vi "MainBootstrap.vi"() -> ()   [LabVIEW 2017]
uses:
  <vilib>/NI/Software Watchdog/Pound/Pound.lvclass
  <vilib>/addons/BlinkProcess/controls/mode.ctl
  <vilib>/addons/InsightCM/Devices/Shared/Common/Controller/controls/operations.ctl
  <vilib>/addons/TraceLogger/TraceLogger.lvlib
  <vilib>/addons/Qbus/Qbus.lvclass
  <vilib>/addons/InsightCM/Devices/Shared/Common/ServerComm/ServerComm.lvlib
  <vilib>/addons/TimerProcess/TimerProcess.lvlib
  <vilib>/addons/BlinkProcess/BlinkProcess.lvlib
  <vilib>/addons/InsightCM/Devices/Shared/Common/TracePointDisplay/TracePointDisplay.lvlib
  <vilib>/addons/InsightCM/Devices/Shared/Common/Controller/Controller.lvlib
  <vilib>/addons/InsightCM/Utilities/GlobalConfiguration/GlobalConfiguration.lvlib
panel:
  out "Log":string
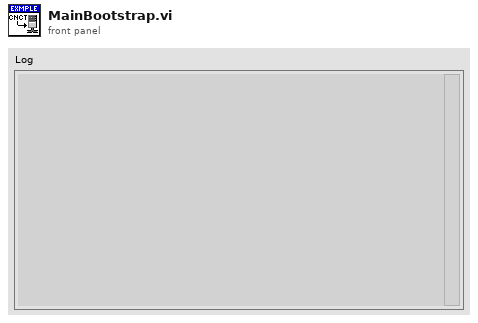
[diagram p1: front panel]
types:
  T1 = typedef "BlinkProcess.lvlib/mode.ctl" = enum16{"Normal", "Error", "On", "Off", "Custom"}
  T2 = typedef "Controller.lvlib/operations.ctl" = enum16{"Unknown", "Startup", "Expected Shutdown"}
  T3 = typedef "ServerComm.lvlib/ConnectionStatus.ctl" = enum16{"Offline", "NotAuthorized", "Online"}
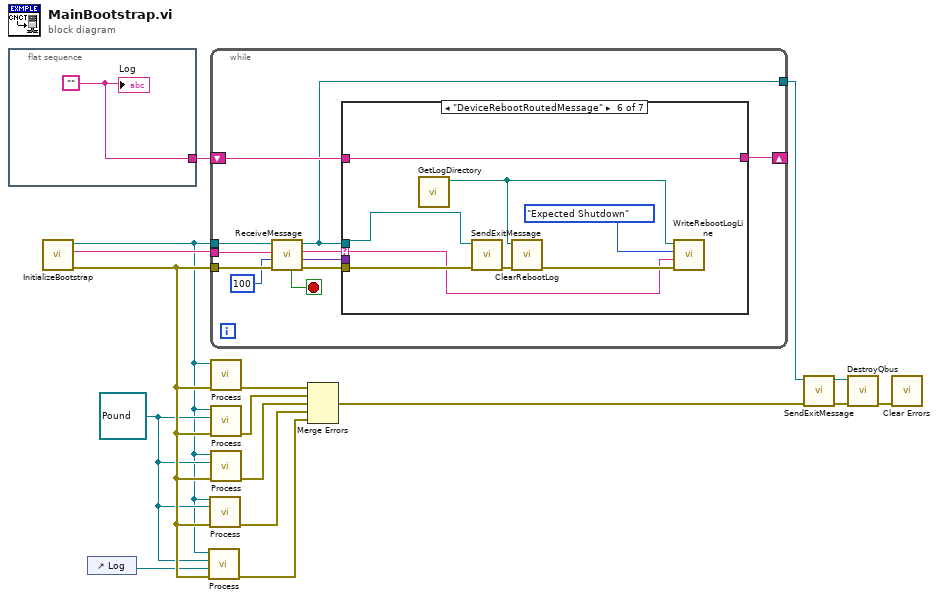
[diagram p0: block diagram]
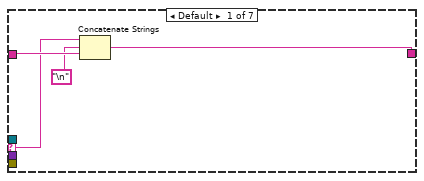
[diagram p2: hidden frame]
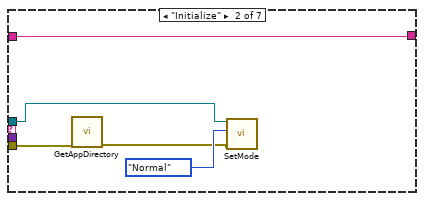
[diagram p3: hidden frame]
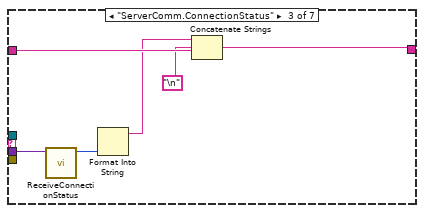
[diagram p4: hidden frame]
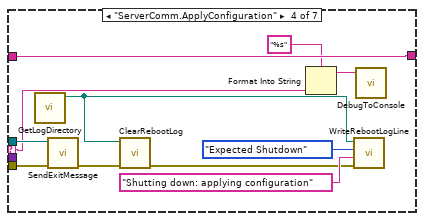
[diagram p5: hidden frame]
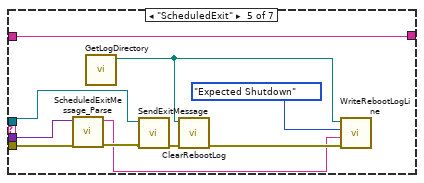
[diagram p6: hidden frame]
diagram:
  w4 = refnum<class "Pound.lvclass"> refnum ("Pound in")
  n1 = flat-sequence {
    tunnel: [w16] -> w13
    frame #0 {
      w16 = ""
      "Log" <- w16
    }
  }
  n2 = call "InitializeBootstrap.vi"() -> ("error out"=w5:errorcluster, "ProcessName"=w7:string, "Qbus out"=w3:refnum<class "Qbus.lvclass">)  [unwired: 9 in]
  n3 = control-ref of="Log"() -> (w1:refnum<vi>)
  n4 = call <vilib>:"Process.vi"("error in (no error)"=w5, "string refnum"=w1, "Pound in"=w4, "Qbus in"=w3) -> ("error out"=w2:errorcluster)  [unwired: 7 in]
  n5 = call <vilib>:"Process.vi"("error in (no error)"=w5, "Pound"=w4, "Qbus in"=w3) -> ("error out"=w6:errorcluster)  [unwired: 8 in]
  n6 = while {
    tunnel: w3 -> [w27]
    tunnel: w7 -> [w26]
    tunnel: w5 -> [w25]
    tunnel: [w20] -> w10
    shift-right: [w18] -> _
    shift-left: w13 -> [w22]
    stop <- w17 stop-if-true
    n7 = call <vilib>:"ReceiveMessage.vi"("error in (no error)"=w25, "timeout (0)"=100, "process name"=w26, "Qbus in"=w27) -> ("error in (no error)"=w19:errorcluster, "message value"=w21:variant, "message name"=w23:string, "Qbus out"=w20:refnum<class "Qbus.lvclass">, "exit"=w17:bool)  [unwired: 2 in, 1 out]
    n8 = case shown="\"DeviceRebootRoutedMessage\"" w23 {
      selector: w23 -> [w29 _ _ w43 _ w64 _]
      tunnel: [w30 w36 w41 w49 w63 w71 w72] -> w18
      tunnel: w22 -> [w31 w36 w42 w49 w63 w71 w72]
      tunnel: w21 -> [_ _ w40 _ w56 _ _]
      tunnel: w20 -> [_ w34 _ w48 w55 w67 _]
      tunnel: w19 -> [_ w33 _ w47 w57 w65 _]
      frame Default {
        n9 = Concatenate Strings(w29, "\n", w31) -> (w30:string)
      }
      frame "Initialize" {
        n10 = call <vilib>:"GetAppDirectory.vi"("error in (no error)"=w33) -> ("error out"=w32:errorcluster)  [unwired: 9 in, 1 out]
        n11 = call <vilib>:"SetMode.vi"("error in (no error)"=w32, "mode"=mode."Normal", "Qbus in"=w34) -> ()  [unwired: 7 in, 2 out]
      }
      frame "ServerComm.ConnectionStatus" {
        n12 = call <vilib>:"ReceiveConnectionStatus.vi"("body"=w40) -> ("status"=w39:T3)  [unwired: 7 in, 3 out]
        n13 = Format Into String(w39) -> (resulting string=w38:string)  [unwired: 3 in, 1 out]
        n14 = Concatenate Strings(w38, "\n", w42) -> (w41:string)
      }
      frame "ServerComm.ApplyConfiguration" {
        n15 = call <vilib>:"GetLogDirectory.vi"() -> ("log dir"=w46:path)  [unwired: 10 in, 1 out]
        n16 = call <vilib>:"SendExitMessage.vi"("error in (no error)"=w47, "Qbus in"=w48) -> ("error in (no error)"=w51:errorcluster)  [unwired: 8 in, 1 out]
        n17 = call <vilib>:"ClearRebootLog.vi"("error in"=w51, "log path"=w46) -> ("error out"=w50:errorcluster)  [unwired: 9 in]
        n18 = Format Into String(format string="%s", w43) -> (resulting string=w44:string)  [unwired: 2 in, 1 out]
        n19 = call <vilib>:"WriteRebootLogLine.vi"("error in"=w50, "reboot log text"="Shutting down: applying configuration", "operation"=operations."Expected Shutdown", "log path"=w46) -> ()  [unwired: 6 in, 2 out]
        n20 = call <vilib>:"DebugToConsole.vi"("String"=w44) -> ()  [unwired: 10 in, 1 out]
      }
      frame "ScheduledExit" {
        n21 = call <vilib>:"ScheduledExitMessage_Parse.vi"("error in (no error)"=w57, "scheduled exit message"=w56) -> ("error out"=w59:errorcluster, "scheduled exit reason"=w58:string)  [unwired: 8 in]
        n22 = call <vilib>:"GetLogDirectory.vi"() -> ("log dir"=w54:path)  [unwired: 10 in, 1 out]
        n23 = call <vilib>:"SendExitMessage.vi"("error in (no error)"=w59, "Qbus in"=w55) -> ("error in (no error)"=w61:errorcluster)  [unwired: 8 in, 1 out]
        n24 = call <vilib>:"ClearRebootLog.vi"("error in"=w61, "log path"=w54) -> ("error out"=w60:errorcluster)  [unwired: 9 in]
        n25 = call <vilib>:"WriteRebootLogLine.vi"("error in"=w60, "reboot log text"=w58, "operation"=operations."Expected Shutdown", "log path"=w54) -> ()  [unwired: 6 in, 2 out]
      }
      frame "DeviceRebootRoutedMessage" {
        n26 = call <vilib>:"GetLogDirectory.vi"() -> ("log dir"=w66:path)  [unwired: 10 in, 1 out]
        n27 = call <vilib>:"SendExitMessage.vi"("error in (no error)"=w65, "Qbus in"=w67) -> ("error in (no error)"=w69:errorcluster)  [unwired: 8 in, 1 out]
        n28 = call <vilib>:"ClearRebootLog.vi"("error in"=w69, "log path"=w66) -> ("error out"=w68:errorcluster)  [unwired: 9 in]
        n29 = call <vilib>:"WriteRebootLogLine.vi"("error in"=w68, "reboot log text"=w64, "operation"=operations."Expected Shutdown", "log path"=w66) -> ()  [unwired: 6 in, 2 out]
      }
      frame "" {
      }
    }
  }
  n30 = call <vilib>:"Process.vi"("error in (no error)"=w5, "qbus in"=w3) -> ("error out"=w15:errorcluster)  [unwired: 9 in]
  n31 = call <vilib>:"Process.vi"("error in (no error)"=w5, "Pound in"=w4, "Qbus in"=w3) -> ("error out"=w14:errorcluster)  [unwired: 8 in]
  n32 = call <vilib>:"Process.vi"("error in (no error)"=w5, "pound in"=w4, "qbus in"=w3) -> ("error out"=w12:errorcluster)  [unwired: 8 in]
  n33 = Merge Errors(w15, w14, w12, w6, w2) -> (w9:errorcluster)
  n34 = call <vilib>:"SendExitMessage.vi"("error in (no error)"=w9, "Qbus in"=w10) -> ("error in (no error)"=w11:errorcluster, "Qbus out"=w8:refnum<class "Qbus.lvclass">)  [unwired: 8 in]
  n35 = call <vilib>:"DestroyQbus.vi"("Qbus"=w8) -> ()  [unwired: 10 in, 1 out]
  n36 = call <vilib>:"Clear Errors.vi"("error in (no error)"=w11) -> ()  [unwired: 5 in, 2 out]
